vi "Sort Into Nested.vi"(8 "error in (no error)":errorcluster, 11 "Found Parent Struct":T1[](array[typedef])) -> (0 "error out":errorcluster, 3 "Nested Structures":T1[](array[typedef]))   [LabVIEW 2023, in "VIDoc Parsing.lvlib" / "Structure Reporter.lvlib"]
uses:
  Structure Reporter.lvlib
  Structure Result 2.ctl
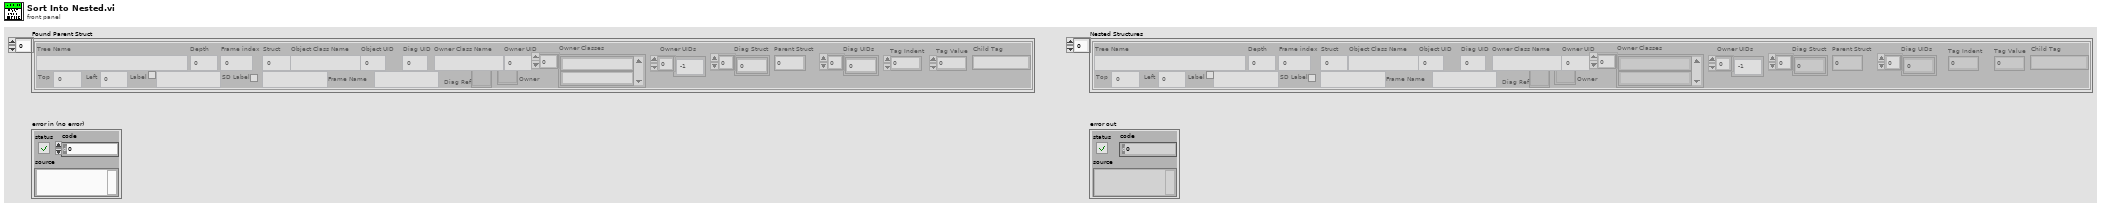
[diagram p1: front panel]
types:
  T1 = typedef "VIDoc Parsing.lvlib/Structure Reporter.lvlib/Structure Result 2.ctl" = cluster{"Depth":i32, "Top":i32, "Left":i32, "Frame index":i32, "Struct":i32, "Object Class Name":string, "Object UID":i32, "Label Visible":bool, "Object Label":string, "SD Label Visible":bool, "Object SD Label":string, "Frame Name":string, "Diag UID":i32, "Owner Class Name":string, "Owner UID":i32, "Diag Struct":i32[], "Parent Struct":i32, "Diag UIDs":i32[], "Tree Name":string, "Diag Ref":refnum<vi>, "Owner Classes":string[], "Owner":refnum<vi>, "Owner UIDs":i32[], "Tag Indent":i32, "Tag Value":i32, "Child Tag":string}
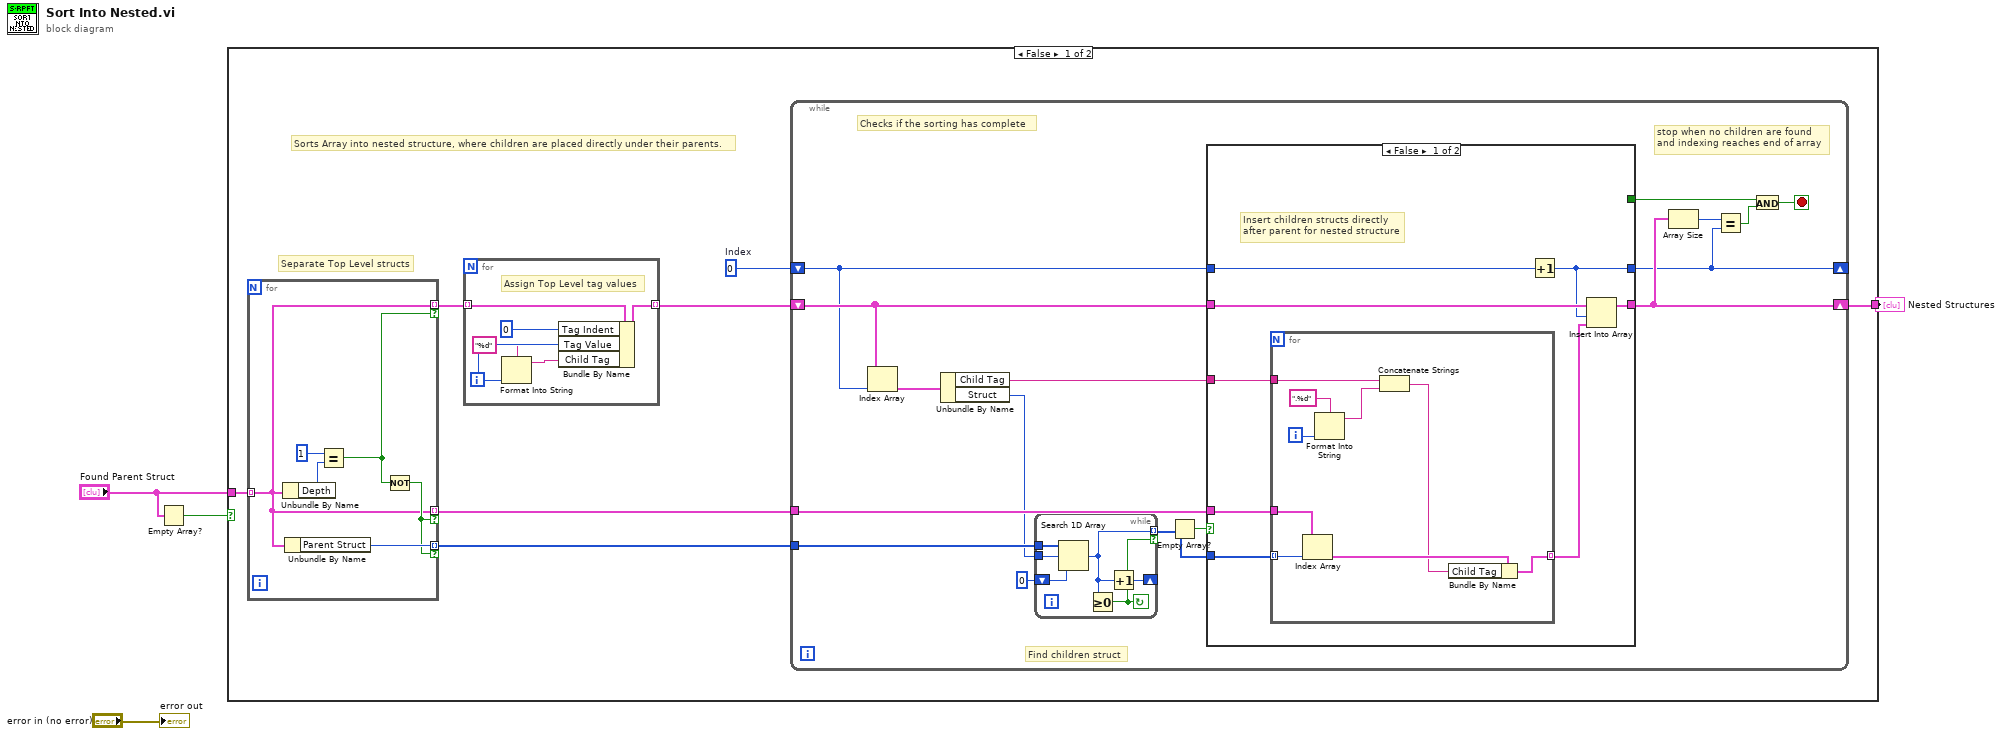
[diagram p0: block diagram]
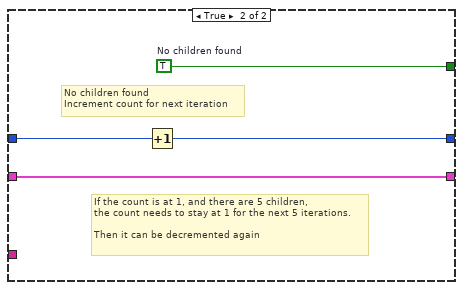
[diagram p2: hidden frame]
diagram:
  n1 = Empty Array?(array="Found Parent Struct") -> (empty?=w1:bool)
  n2 = case shown="False" w1 {
    tunnel: [w10 _] -> w4
    tunnel: "Found Parent Struct" -> [w5 _]
    frame False {
      w11 = 0  # Index
      # "Sorts Array into nested structure, where children are placed directly under their parents."
      # "Separate Top Level structs"
      n3 = for {
        tunnel: w5 -> [w61] mode=indexing
        tunnel: [w61] -> w8 mode=indexing if=w64
        tunnel: [w61] -> w6 mode=indexing if=w62
        tunnel: [w63] -> w7 mode=indexing if=w62
        n4 = Unbundle By Name(w61) -> ("Depth"=w66:i32)
        n5 = Unbundle By Name(w61) -> ("Parent Struct"=w63:i32)
        n6 = Equal?(x=1, y=w66) -> (x = y?=w64:bool)
        n7 = Not(x=w64) -> (.not. x?=w62:bool)
      }
      n8 = for {
        tunnel: w8 -> [w59] mode=indexing
        tunnel: [w58] -> w9 mode=indexing
        i -> [w57]
        # "Assign Top Level tag values"
        n9 = Format Into String(format string="%d", w57) -> (resulting string=w55:string)  [unwired: 2 in, 1 out]
        n10 = Bundle By Name(cluster=w59, "Tag Indent"=0, "Tag Value"=w57, "Child Tag"=w55) -> (w58:T1)
      }
      n11 = while {
        tunnel: w6 -> [w26]
        tunnel: w7 -> [w14]
        shift-right: [w17] -> _
        shift-left: w11 -> [w23]
        shift-right: [w18] -> w10
        shift-left: w9 -> [w24]
        stop <- w19 stop-if-true
        # "stop when no children are found \nand indexing reaches end of array"
        # "Find children struct"
        # "Checks if the sorting has complete"
        n12 = Index Array(array=w24, index=w23) -> (element=w27:T1)
        n13 = Unbundle By Name(w27) -> ("Child Tag"=w16:string, "Struct"=w13:i32)
        n14 = while {
          shift-right: [w30] -> _
          shift-left: 0 ("Start Index (0)") -> [w33]
          tunnel: w14 -> [w32]
          tunnel: w13 -> [w31]
          tunnel: [w29] -> w12 mode=indexing if=w28
          stop <- w28 continue-if-true
          n15 = Search 1D Array(1D array=w32, element=w31, start index (0)=w33) -> (index of element=w29:i32)
          n16 = Greater Or Equal To 0?(x=w29) -> (x >= 0?=w28:bool)
          n17 = Increment(x=w29) -> (x+1=w30:i32)
        }
        n18 = Empty Array?(array=w12) -> (empty?=w25:bool)
        n19 = case shown="False" w25 {
          tunnel: w26 -> [w41 _]
          tunnel: w12 -> [w40 _]
          tunnel: w24 -> [w39 w54]
          tunnel: w23 -> [w36 w53]
          tunnel: [w37 w54] -> w18
          tunnel: [_ w52] -> w21
          tunnel: [w35 w51] -> w17
          tunnel: w16 -> [w34 _]
          frame False {
            # "Insert children structs directly\nafter parent for nested structure"
            n20 = for {
              tunnel: w41 -> [w50]
              tunnel: w40 -> [w49] mode=indexing
              tunnel: [w47] -> w38 mode=indexing
              tunnel: w34 -> [w43]
              i -> [w46]
              n21 = Index Array(array=w50, index=w49) -> (element=w48:T1)
              n22 = Format Into String(format string=".%d", w46) -> (resulting string=w44:string)  [unwired: 2 in, 1 out]
              n23 = Concatenate Strings(w43, w44) -> (w42:string)
              n24 = Bundle By Name(cluster=w48, "Child Tag"=w42) -> (w47:T1)
            }
            n25 = Increment(x=w36) -> (x+1=w35:i32)
            n26 = Insert Into Array(array=w39, index=w35, new element=w38) -> (w37:T1[])
          }
          frame True {
            w52 = TRUE  # No children found
            # "If the count is at 1, and there are 5 children,\nthe count needs to stay at 1 for the next 5 iterations.\n\nThen it can be decremented again"
            # "No children found\nIncrement count for next iteration"
            n27 = Increment(x=w53) -> (x+1=w51:i32)
          }
        }
        n28 = Array Size(array=w18) -> (size(s)=w22:i32)
        n29 = Equal?(x=w22, y=w17) -> (x = y?=w20:bool)
        n30 = And(x=w21, y=w20) -> (x .and. y?=w19:bool)
      }
    }
    frame True {
    }
  }
  "Nested Structures" <- w4
  "error out" <- "error in (no error)"
